vi "Custom.vi"(8 "error in (no error)":errorcluster) -> (0 "error out":errorcluster={"status"=FALSE, "code"=1073676294, "source"="VISA Read in SerialCommunicationTransport.vi"})   [LabVIEW 2020, in "FirmataClient.lvlib"]
doc: "Allows sending custom messages to the board. Enter the message as hex separated with \"-\" (i.e. to request firrmware, enter \"F0-79-F7\" and expect \"F0-79-2-5-53-0-74-0-61-0-6E-0-64-0-61-0-72-0-64-0-46-0-69-0-72-0-6D-0-61-0-74-0-61-0-2E-0-69-0-6E-0-6F-0-F7\" as \"StandardFirmata.ino and v2.5\")."
uses:
  FirmataClient.lvlib
  Transports/Controls/Transport Commands.ctl
panel:
  in  "Message In":string="F0-79-F7"
  out "Response":string="F0-79-2-5-53-0-74-0-61-0-6E-0-64-0-61-0-72-0-64-0-46-0-69-0-72-0-6D-0-61-0-74-0-61-0-2E-0-69-0-6E-0-6F-0-F7\r\n"
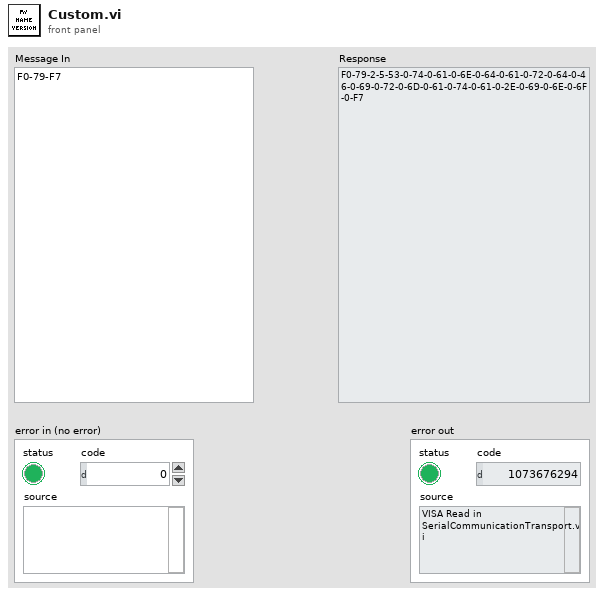
[diagram p1: front panel]
types:
  T1 = typedef "Transport Commands.ctl" = enum16{"Initialize", "Transmit - Receive", "Cleanup", "Cleanup And Stop"}
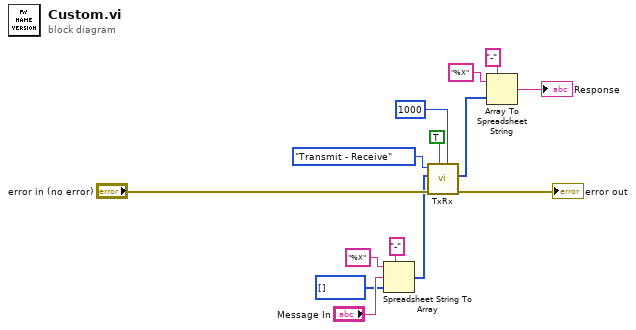
[diagram p0: block diagram]
diagram:
  n1 = Spreadsheet String To Array(delimiter (Tab)="-", format string="%X", spreadsheet string="Message In", array type (2D Dbl)=u8[] []) -> (array=w6:u8[])
  n2 = call "TxRx.vi"("Reply Timeout Ms"=1000, "Wait For Reply?"=TRUE, "error in"="error in (no error)", "Message"=w6, "Command"=Transport_Commands."Transmit - Receive") -> ("error out"=→"error out":errorcluster, "Reply"=w3:u8[])  [unwired: 5 in]
  n3 = Array To Spreadsheet String(delimiter (Tab)="-", array=w3, 3:"%X" ("format string")) -> (spreadsheet string=→"Response":string)
